vi "SubVI_ALD-Process-Step_Purge_V16.vi"(0 "error in (no error)":errorcluster, 1 "Mod8 DAQ Name":tag, 2 "Mod7 DAQ Name":tag, 3 "Purge Array":T2={"Mod7"=[FALSE, FALSE, FALSE, FALSE, FALSE, FALSE, FALSE, FALSE], "Mod8"=[FALSE, FALSE, FALSE, FALSE, FALSE, FALSE, FALSE, FALSE]}, 5 "Total # Steps":i32, 7 "Purge Time (sec)":dbl, 12 "ProcessStep Input Cluster":T1, 14 "Recipe Step \nNumber":i32) -> (4 "error out":errorcluster, 8 "Purge Start Timestamp":timestamp, 15 "Execution Aborted \nDuring This Recipe Step?":bool)   [LabVIEW 2026]
uses:
  CTRL_DO Boolean Array Cluster_V16.ctl
panel:
  out "Purge Start Time":dbl
  # "NEED TO UPDATE SUBVI DESCRIPTION"
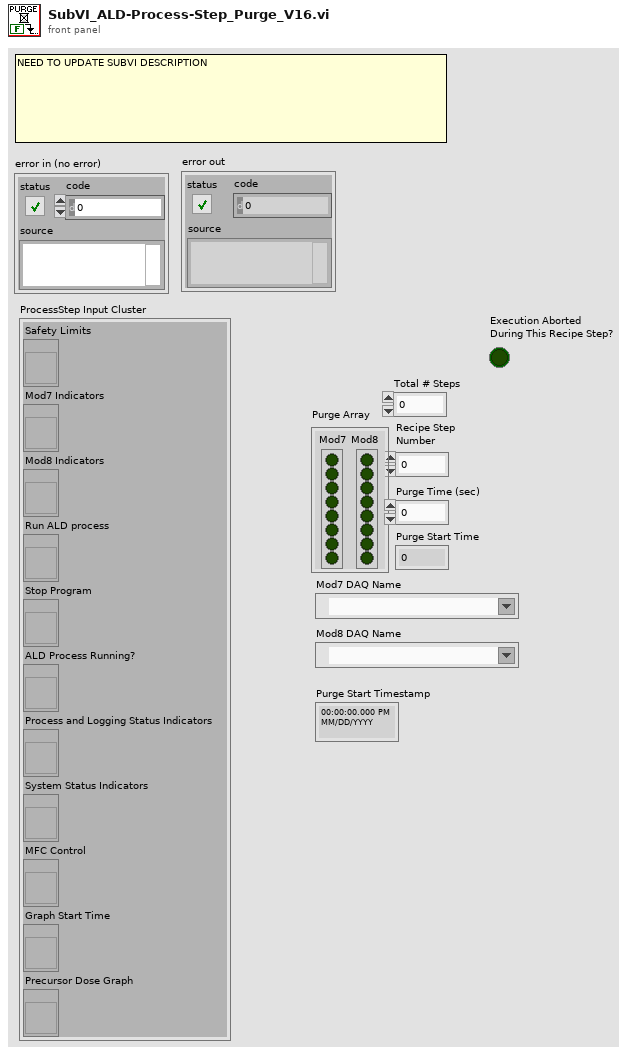
[diagram p1: front panel]
types:
  T1 = cluster{"Safety Limits":refnum<vi>, "Mod7 Indicators ":refnum<vi>, "Mod8 Indicators":refnum<vi>, "Run ALD process":refnum<vi>, "Stop Program":refnum<vi>, "ALD Process Running?":refnum<vi>, "Process and Logging Status Indicators":refnum<vi>, "System Status Indicators":refnum<vi>, "MFC Control":refnum<vi>, "Graph Start Time":refnum<vi>, "Precursor Dose Graph":refnum<vi>}
  T2 = typedef "CTRL_DO Boolean Array Cluster_V16.ctl" = cluster{"Mod7":bool[], "Mod8":bool[]}
  T3 = typedef "CTRL_ProcessLoggingStatusIndicator_V14.ctl" = cluster{"ALD Process Status:":string, "Logging Data to:":path, "Process Start Time:":string, "Process End Time:":string, "Steps Completed:":string}
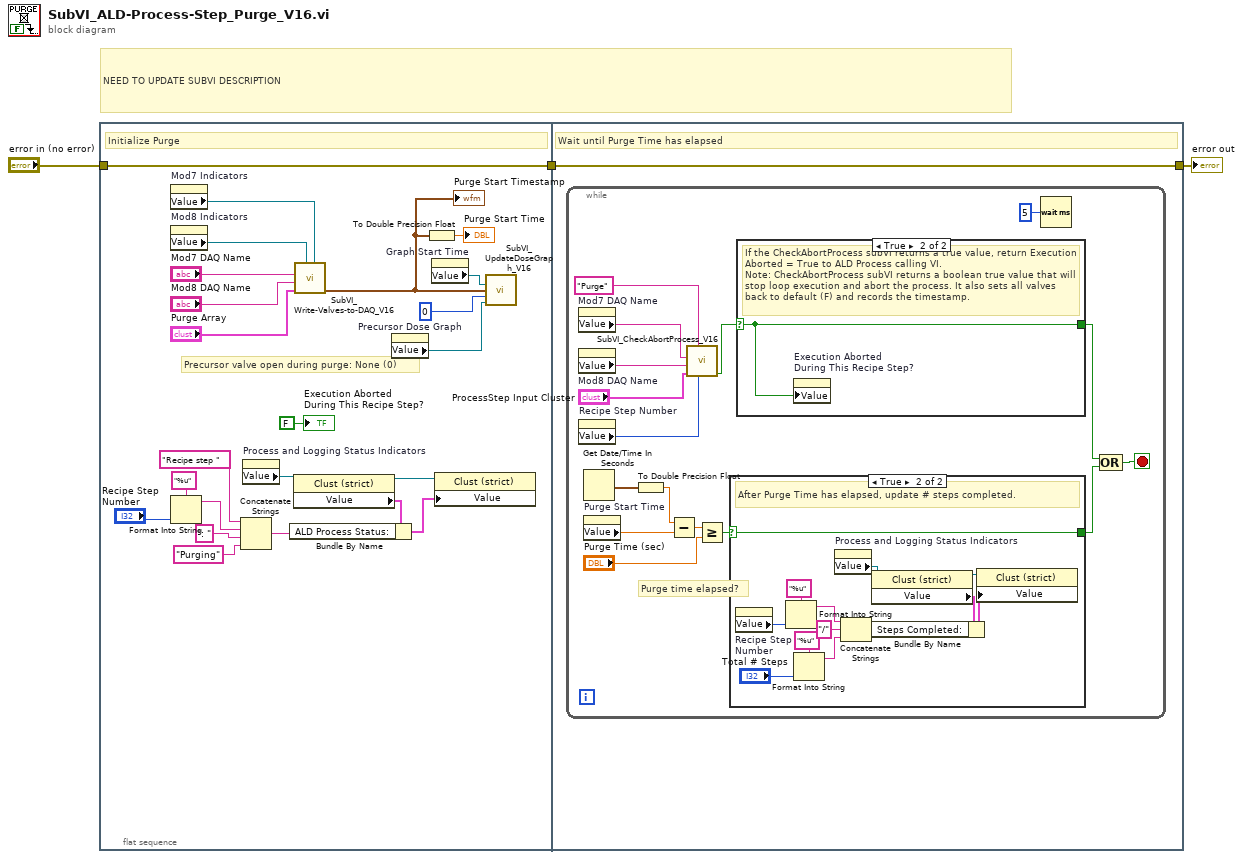
[diagram p0: block diagram]
diagram:
  # "NEED TO UPDATE SUBVI DESCRIPTION"
  n1 = flat-sequence {
    tunnel: "error in (no error)" -> [w25]
    tunnel: [w25] -> w1
    tunnel: [w27] -> w2
    tunnel: w1 -> [w27]
    frame #0 {
      # "Precursor valve open during purge: None (0)"
      # "Initialize Purge"
      n2 = property on="Mod7 Indicators" class="LVObjRef (strict)"() -> ("Value"=w9:refnum<vi>)  [unwired: 2 in, 2 out]
      n3 = property on="Mod8 Indicators" class="LVObjRef (strict)"() -> ("Value"=w10:refnum<vi>)  [unwired: 2 in, 2 out]
      n4 = Format Into String(format string="%u", "Recipe Step \nNumber") -> (resulting string=w20:string)  [unwired: 2 in, 1 out]
      n5 = Concatenate Strings("Recipe step ", w20, ": " ("string"), "Purging" ("Value")) -> (w23:string)
      n6 = property on="Process and Logging Status Indicators" class="LVObjRef (strict)"() -> ("Value"=w14:refnum<vi>)  [unwired: 2 in, 2 out]
      n7 = property class="Clust (strict)"(reference=w14) -> (reference out=w15:refnum<vi>, "Value"=w16:T3)  [unwired: 1 in, 1 out]
      n8 = Bundle By Name(cluster=w16, "ALD Process Status:"=w23) -> (w17:T3)
      n9 = call "SubVI_Write-Valves-to-DAQ_V16.vi"("Mod7 Indicators Ref"=w9, "Mod8 Indicators Ref"=w10, "DO Boolean Array Cluster"="Purge Array", "Mod8 Port Name"="Mod8 DAQ Name", "Mod7 Port Name"="Mod7 DAQ Name") -> ("current time"=w5:timestamp)  [unwired: 3 in, 3 out]
      "Purge Start Timestamp" <- w5
      n10 = property on="Precursor Dose Graph" class="LVObjRef (strict)"() -> ("Value"=w13:refnum<vi>)  [unwired: 2 in, 2 out]
      n11 = To Double Precision Float(number=w5) -> (double precision float=→"Purge Start Time":dbl)
      n12 = property on="Graph Start Time" class="LVObjRef (strict)"() -> ("Value"=w11:refnum<vi>)  [unwired: 2 in, 2 out]
      n13 = property class="Clust (strict)"(reference=w15, "Value"=w17) -> ()  [unwired: 1 in, 2 out]
      n14 = call "SubVI_UpdateDoseGraph_V16.vi"("Graph Start Time"=w11, "New Timestamp"=w5, "Precursor Valve Open"=0 ("Precursor"), "Precursor Dose Graph"=w13) -> ()  [unwired: 11 in, 1 out]
      "Execution Aborted \nDuring This Recipe Step?" <- FALSE ("Execution Aborted?")
    }
    frame #1 {
      # "Wait until Purge Time has elapsed"
      n15 = while {
        stop <- w42 stop-if-true
        # "Purge time elapsed?"
        n16 = property on="Mod7 DAQ Name" class="DAQmxName"() -> ("Value"=w33:string)  [unwired: 2 in, 2 out]
        n17 = property on="Mod8 DAQ Name" class="DAQmxName"() -> ("Value"=w32:string)  [unwired: 2 in, 2 out]
        n18 = property on="Recipe Step Number" class="DigNum (strict)"() -> ("Value"=w31:i32)  [unwired: 2 in, 2 out]
        n19 = Get Date/Time In Seconds() -> (seconds since 1Jan1904=w28:timestamp)
        n20 = property on="Purge Start Time" class="DigNum (strict)"() -> ("Value"=w36:dbl)  [unwired: 2 in, 2 out]
        n21 = To Double Precision Float(number=w28) -> (double precision float=w37:dbl)
        n22 = Subtract(x=w37, y=w36) -> (x-y=w35:dbl)
        n23 = call "SubVI_CheckAbortProcess_V16.vi"("Process Step"=w31, "Step Description"="Purge", "ProcessStep Input Cluster"="ProcessStep Input Cluster", "Mod8 DAQ Name"=w32, "Mod7 DAQ Name"=w33) -> ("Abort Process Execution"=w39:bool)  [unwired: 5 in, 1 out]
        n24 = Greater Or Equal?(x=w35, y="Purge Time (sec)") -> (x >= y?=w34:bool)
        n25 = case shown="True" w34 {
          selector: w34 -> [w44 w51]
          tunnel: [w44 w51] -> w40
          frame False {
            # "Wait until Purge Time has elapsed."
          }
          frame True {
            # "After Purge Time has elapsed, update # steps completed."
            n26 = property on="Recipe Step \nNumber" class="DigNum (strict)"() -> ("Value"=w53:i32)  [unwired: 2 in, 2 out]
            n27 = Format Into String(format string="%u", w53) -> (resulting string=w48:string)  [unwired: 2 in, 1 out]
            n28 = Format Into String(format string="%u", "Total # Steps") -> (resulting string=w46:string)  [unwired: 2 in, 1 out]
            n29 = property on="Process and Logging Status Indicators" class="LVObjRef (strict)"() -> ("Value"=w57:refnum<vi>)  [unwired: 2 in, 2 out]
            n30 = Concatenate Strings(w48, "/" ("string"), w46) -> (w45:string)
            n31 = property class="Clust (strict)"(reference=w57) -> (reference out=w56:refnum<vi>, "Value"=w55:T3)  [unwired: 1 in, 1 out]
            n32 = Bundle By Name(cluster=w55, "Steps Completed:"=w45) -> (w54:T3)
            n33 = property class="Clust (strict)"(reference=w56, "Value"=w54) -> ()  [unwired: 1 in, 2 out]
          }
        }
        n34 = case shown="True" w39 {
          selector: w39 -> [w58 w59]
          tunnel: [w58 w59] -> w41
          frame False {
            # "If the CheckAbortProcess subVI returns a false value, wait until Purge Time has elapsed."
          }
          frame True {
            # "If the CheckAbortProcess subVI returns a true value, return Execution Aborted = True to ALD Process calling VI. \nNote: CheckAbortProcess subVI returns a boolean true value that will stop loop execution and abort the process. It also sets all valves back to default (F) and records the timestamp."
            n35 = property on="Execution Aborted \nDuring This Recipe Step?" class="Bool (strict)"("Value"=w59) -> ()  [unwired: 2 in, 2 out]
          }
        }
        n36 = Wait (ms)(milliseconds to wait=u32 5) -> ()  [unwired: 1 out]
        n37 = Compound Arithmetic op=OR(w41, w40) -> (w42:bool)
      }
    }
  }
  "error out" <- w2
